vi "Replace Missing Denpendency VIs - Client Wrapper.vi"(8 "error in":errorcluster, 10 "gRPC Service Name":string, 11 "PluginGenerator_MetaDataObj":refnum<class "PluginGenerator_MetaDataObj.lvclass">) -> (0 "error out":errorcluster, 3 "PluginGenerator_MetaDataObj out":refnum<class "PluginGenerator_MetaDataObj.lvclass">)   [LabVIEW 2021, in "Plugin Generator.lvlib"]
uses:
  Plugin Generator.lvlib
  PluginGenerator_MetaDataObj/PluginGenerator_MetaDataObj.lvclass
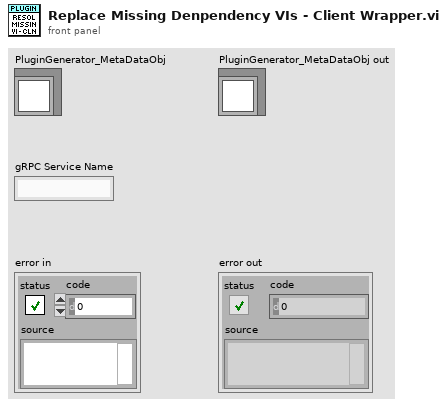
[diagram p1: front panel]
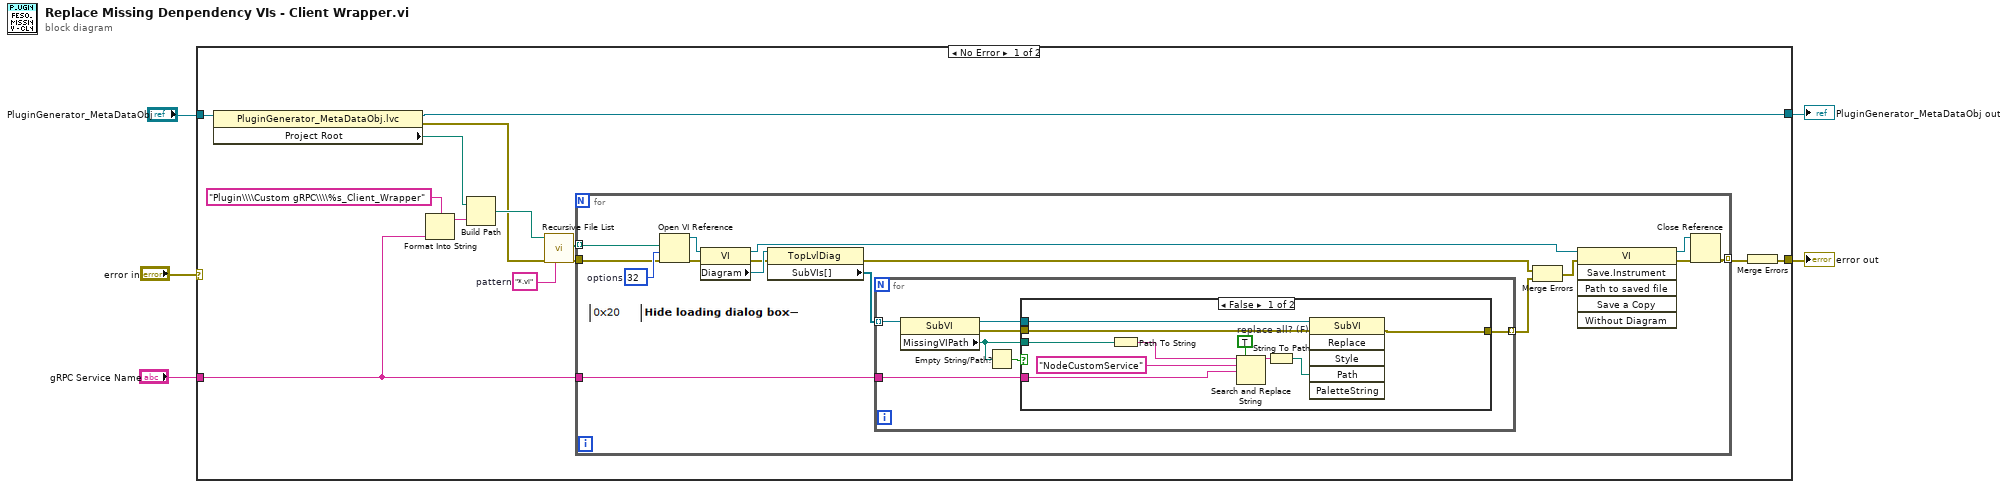
[diagram p0: block diagram]
diagram:
  n1 = case shown="No Error" "error in" {
    selector: "error in" -> [_ w53]
    tunnel: [w12 w53] -> w5
    tunnel: "gRPC Service Name" -> [w11 _]
    tunnel: "PluginGenerator_MetaDataObj" -> [w10 w54]
    tunnel: [w6 w54] -> w1
    frame No Error {
      w17 = "*.vi"  # pattern
      n2 = property class="PluginGenerator_MetaDataObj.lvc"(reference=w10) -> (reference out=w6:refnum<class "PluginGenerator_MetaDataObj.lvclass">, error out=w9:errorcluster, "Project Root"=w8:path)  [unwired: 1 in]
      n3 = Format Into String(format string="Plugin\\\\Custom gRPC\\\\%s_Client_Wrapper" ("Class Name"), w11) -> (resulting string=w16:string)  [unwired: 2 in, 1 out]
      n4 = Build Path(base path=w8, name or relative path=w16) -> (appended path=w15:path)
      n5 = call <vilib>:"Recursive File List.vi"("pattern"=w17, "error in (no error)"=w9, "Folder Path"=w15) -> ("error out"=w7:errorcluster, "All Files in Dir"=w18:path[])  [unwired: 4 in, 3 out]
      n6 = for {
        tunnel: w18 -> [w34] mode=indexing
        tunnel: w11 -> [w29]
        tunnel: [w26] -> w13 mode=indexing
        tunnel: w7 -> [w24]
        w25 = 32  # options
        n7 = Open VI Reference(vi path=w34, options=w25, error in (no error)=w24) -> (vi reference=w33:refnum<vi>, error out=w27:errorcluster)  [unwired: 3 in]
        n8 = property class="VI"(reference=w33, error in=w27) -> (reference out=w31:refnum<vi>, error out=w28:errorcluster, "Diagram"=w32:refnum<vi>)
        n9 = property class="TopLvlDiag"(reference=w32, error in=w28) -> (error out=w19:errorcluster, "SubVIs[]"=w30:refnum<vi>[])  [unwired: 1 out]
        n10 = for {
          tunnel: w30 -> [w41] mode=indexing
          tunnel: w29 -> [w37]
          tunnel: [w35] -> w20 mode=indexing
          n11 = property class="SubVI"(reference=w41) -> (reference out=w39:refnum<vi>, error out=w36:errorcluster, "MissingVIPath"=w38:path)  [unwired: 1 in]
          n12 = Empty String/Path?(string/path=w38) -> (empty?=w40:bool)
          n13 = case shown="False" w40 {
            tunnel: w39 -> [w51 _]
            tunnel: w38 -> [w49 _]
            tunnel: w37 -> [w45 _]
            tunnel: w36 -> [w43 w52]
            tunnel: [w42 w52] -> w35
            frame False {
              w44 = TRUE  # replace all? (F)
              n14 = Path To String(path=w49) -> (string=w50:string)
              n15 = Search and Replace String(replace all?=w44, input string=w50, search string="NodeCustomService", replace string=w45) -> (result string=w47:string)  [unwired: 4 in, 3 out]
              n16 = String To Path(string=w47) -> (path=w46:path)
              n17 = invoke class="SubVI" method="Replace"(reference=w51, error in=w43, "Path"=w46) -> (error out=w42:errorcluster)  [unwired: 3 in, 5 out]
            }
            frame True {
            }
          }
        }
        n18 = Merge Errors(w19, w20) -> (w21:errorcluster)
        n19 = invoke class="VI" method="Save.Instrument"(reference=w31, error in=w21) -> (reference out=w23:refnum<vi>, error out=w22:errorcluster)  [unwired: 4 in, 4 out]
        n20 = Close Reference(reference=w23, error in (no error)=w22) -> (error out=w26:errorcluster)
      }
      n21 = Merge Errors(w13) -> (w12:errorcluster)
    }
    frame Error {
    }
  }
  "error out" <- w5
  "PluginGenerator_MetaDataObj out" <- w1
